vi "swapArrayElement.vi"(8 "Array":dbl[](array[numeric]), 9 "Index 2":i32, 10 "Index 1":i32, 11 "swap":bool) -> (3 "Swapped Array":dbl[](array[numeric]))   [LabVIEW 2014]
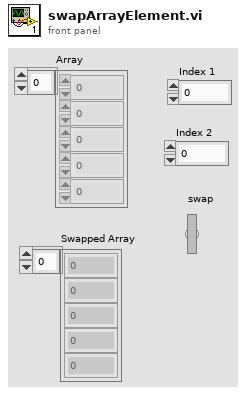
[diagram p1: front panel]
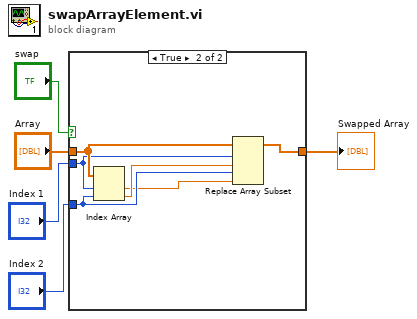
[diagram p0: block diagram]
diagram:
  n1 = case shown="True" "swap" {
    tunnel: "Array" -> [w6 w12]
    tunnel: "Index 1" -> [_ w11]
    tunnel: "Index 2" -> [_ w9]
    tunnel: [w6 w7] -> w2
    frame False {
    }
    frame True {
      n2 = Index Array(array=w12, index #1=w11, index #2=w9) -> (element #1=w8:dbl, element #2=w10:dbl)
      n3 = Replace Array Subset(array=w12, new element #1=w10, index #1=w11, new element #2=w8, index #2=w9) -> (w7:dbl[])
    }
  }
  "Swapped Array" <- w2
